vi "Write Autotest_Result Msg.vi"(10 "Actor_Autotest.lvlib:Autotest_Result Msg.lvclass":refnum<class "Autotest_Result Msg.lvclass">, 11 "Actor_Autotest in":refnum<class "Actor_Autotest.lvclass">) -> (3 "Actor_Autotest out":refnum<class "Actor_Autotest.lvclass">)   [LabVIEW 2020, in "Library Core.lvlib" / "Actor_Autotest.lvlib" / "Actor_Autotest.lvclass"]
uses:
  Actor_Autotest.lvclass
  Actor_Autotest Messages/Autotest_Result Msg/Autotest_Result Msg.lvclass
  Actor_Autotest.lvclass/Actor_Autotest.ctl
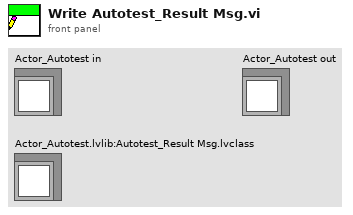
[diagram p1: front panel]
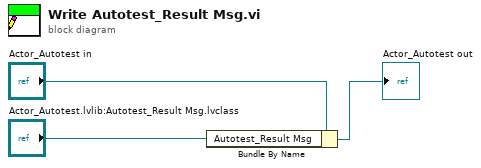
[diagram p0: block diagram]
diagram:
  n1 = Bundle By Name(cluster="Actor_Autotest in", "Autotest_Result Msg"="Actor_Autotest.lvlib:Autotest_Result Msg.lvclass") -> (→"Actor_Autotest out":refnum<class "Actor_Autotest.lvclass">)
